vi "TwGetSumSpectrumFromShMem.vi"(2 "Normalize":bool, 3 "SumSpectrum in":dbl[](array[numeric]), 4 "error in (no error)":errorcluster) -> (0 "SumSpectrum out":dbl[](array[numeric]), 1 "error out":errorcluster)   [LabVIEW 2009]
uses:
  TofDaqDll.dll
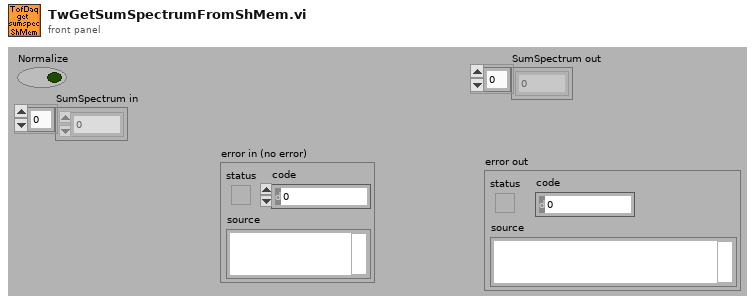
[diagram p1: front panel]
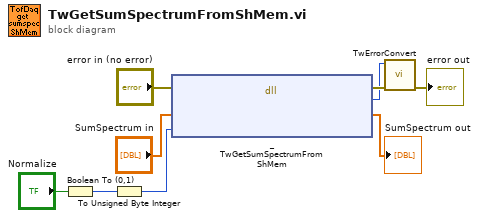
[diagram p0: block diagram]
diagram:
  n1 = Boolean To (0,1)(Boolean="Normalize") -> (0, 1=w5:i16)
  n2 = To Unsigned Byte Integer(number=w5) -> (unsigned 8bit integer=w4:u8)
  n3 = dll-call lib="C:/Users/TofEmp/Desktop/LVTest/TofDaqDll.dll" fn="_TwGetSumSpectrumFromShMem"(error in="error in (no error)", "Spectrum"="SumSpectrum in", "Normalize"=w4) -> (error out=w8:errorcluster, "TwRetVal"=w7:i32, "Spectrum"=→"SumSpectrum out":dbl[])  [unwired: 3 in, 1 out]
  n4 = call "TwErrorConvert.vi"("error in (no error)"=w8, "error code"=w7) -> ("error out"=→"error out":errorcluster)  [unwired: 9 out]
